vi "Qn5_X.vi"(11 "String":string) -> (3 "Qn":dbl[](array[numeric]))   [LabVIEW 2015]
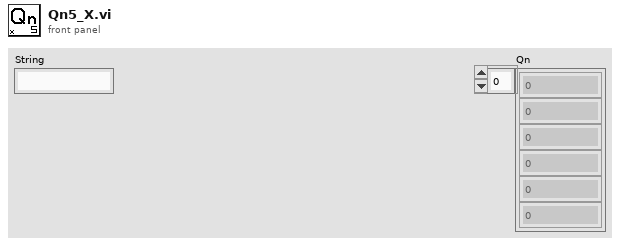
[diagram p1: front panel]
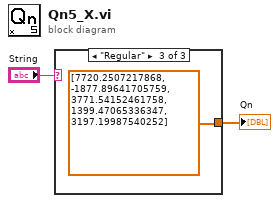
[diagram p0: block diagram]
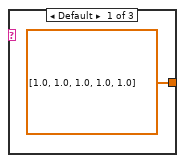
[diagram p2: hidden frame]
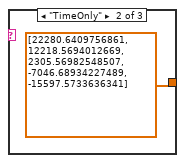
[diagram p3: hidden frame]
diagram:
  n1 = case shown="\"Regular\"" "String" {
    tunnel: [dbl[] [1.0, 1.0, 1.0, 1.0, 1.0] ("Qn") dbl[] [22280.6409756861, 12218.5694012669, 2305.56982548507, -7046.68934227489, -15597.5733636341] ("Qn") dbl[] [7720.2507217868, -1877.89641705759, 3771.54152461758, 1399.47065336347, 3197.19987540252] ("Qn")] -> w1
    frame Default {
    }
    frame "TimeOnly" {
    }
    frame "Regular" {
    }
  }
  "Qn" <- w1
